vi "PV_TimeSyncClient_Test.vi"() -> ()   [LabVIEW 2019]
uses:
  <vilib>/Rock Robotics/WPI/ThirdParty/PhotonVisionLib/SubVI/PhotonVision_Globals.vi
  <vilib>/Rock Robotics/WPI/ThirdParty/PhotonVisionLib/PhotonVisionLib.lvlib
panel:
  out "PV_TimeSyncClientWriteErrClus":errorcluster
  out "PV_TimeSyncClientReadErrClus":errorcluster
  out "PV_TimeSyncClientLastRcvTime":i64
  out "PV_TimeSyncClientLastRcvVer":i8
  out "PV_TimeSyncClientLastSentTime":i64
  out "PV_TimeSyncClientLoopCnt":i32
  out "PV_TimeSyncClientReadErr":bool
  out "PV_TimeSyncClientStop":bool
  out "PV_TimeSyncClientTimeOffset":i64
  out "PV_TimeSyncClientWriteErr":bool
  out "PV_TimeSyncClientLastRcvId":i8
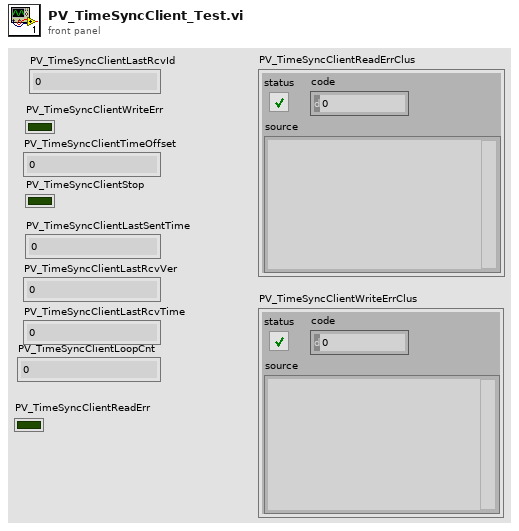
[diagram p1: front panel]
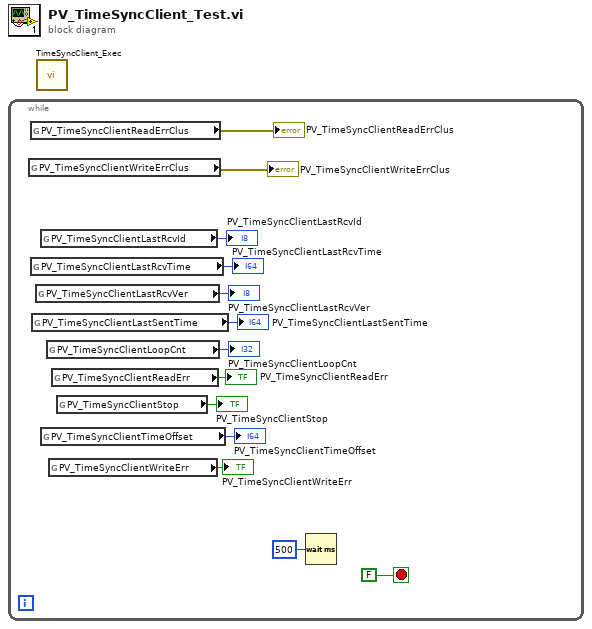
[diagram p0: block diagram]
diagram:
  n1 = while {
    stop <- FALSE stop-if-true
    n2 = global read "PhotonVision_Globals.vi" "PV_TimeSyncClientWriteErrClus"() -> (→"PV_TimeSyncClientWriteErrClus":errorcluster)
    n3 = global read "PhotonVision_Globals.vi" "PV_TimeSyncClientReadErrClus"() -> (→"PV_TimeSyncClientReadErrClus":errorcluster)
    n4 = global read "PhotonVision_Globals.vi" "PV_TimeSyncClientLastRcvTime"() -> (→"PV_TimeSyncClientLastRcvTime":i64)
    n5 = global read "PhotonVision_Globals.vi" "PV_TimeSyncClientLastSentTime"() -> (→"PV_TimeSyncClientLastSentTime":i64)
    n6 = global read "PhotonVision_Globals.vi" "PV_TimeSyncClientLastRcvVer"() -> (→"PV_TimeSyncClientLastRcvVer":i8)
    n7 = global read "PhotonVision_Globals.vi" "PV_TimeSyncClientLastRcvId"() -> (→"PV_TimeSyncClientLastRcvId":i8)
    n8 = global read "PhotonVision_Globals.vi" "PV_TimeSyncClientTimeOffset"() -> (→"PV_TimeSyncClientTimeOffset":i64)
    n9 = global read "PhotonVision_Globals.vi" "PV_TimeSyncClientLoopCnt"() -> (→"PV_TimeSyncClientLoopCnt":i32)
    n10 = global read "PhotonVision_Globals.vi" "PV_TimeSyncClientWriteErr"() -> (→"PV_TimeSyncClientWriteErr":bool)
    n11 = global read "PhotonVision_Globals.vi" "PV_TimeSyncClientReadErr"() -> (→"PV_TimeSyncClientReadErr":bool)
    n12 = global read "PhotonVision_Globals.vi" "PV_TimeSyncClientStop"() -> (→"PV_TimeSyncClientStop":bool)
    n13 = Wait (ms)(milliseconds to wait=u32 500) -> ()  [unwired: 1 out]
  }
  n14 = call <vilib>:"TimeSyncClient_Exec.vi"() -> ()  [unwired: 12 in]
